vi "Check_Particle_State_NextTime_Roadblock.vi"(0 "Particle State at T":T3(array[cluster]), 1 "Torque?":bool, 2 "Torque":dbl, 3 "Rot diffusion\nfor Cargo?":bool, 5 "Tau_On":i32, 7 "Tau_Off":i32, 9 "Posi_Roadblock":dbl[][](array[numeric]), 11 "Center State at T":T1, 12 "Asymmetry (X, Y)":dbl[](array[numeric]), 13 "SD":dbl, 14 "Rot diffusion\nfor Cargo":dbl format="%#_13g") -> (4 "Particle State at T+1":T2(array[cluster]), 15 "New Center State at T":T1)   [LabVIEW 2020]
uses:
  <vilib>/gmath/statdist.llb/Normal Random.vi
  <vilib>/gmath/NI_Gmath.lvlib
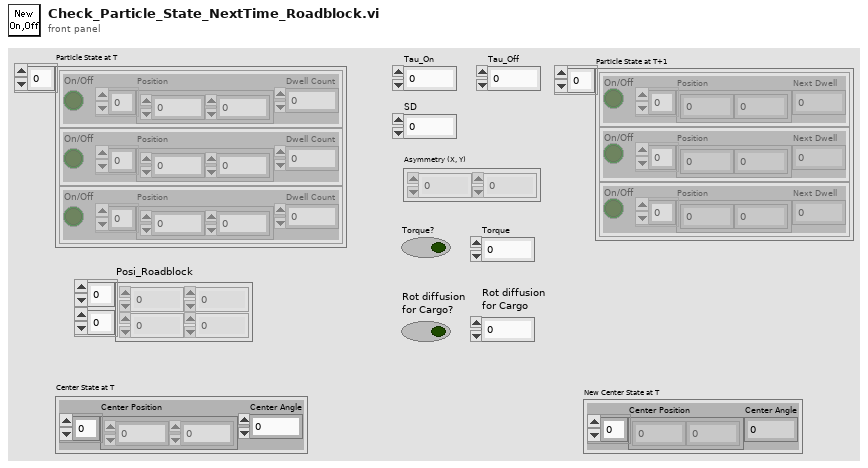
[diagram p1: front panel]
types:
  T1 = cluster{"Center Position":dbl[], "Center Angle":dbl}
  T2 = cluster{"On/Off":bool, "Position":dbl[], "Next Dwell":i32}[]
  T3 = cluster{"On/Off":bool, "Position":dbl[], "Dwell Count":i32}[]
  T4 = cluster{"On/Off":bool, "Hinderance posi":dbl[], "Next Dwell":i32}
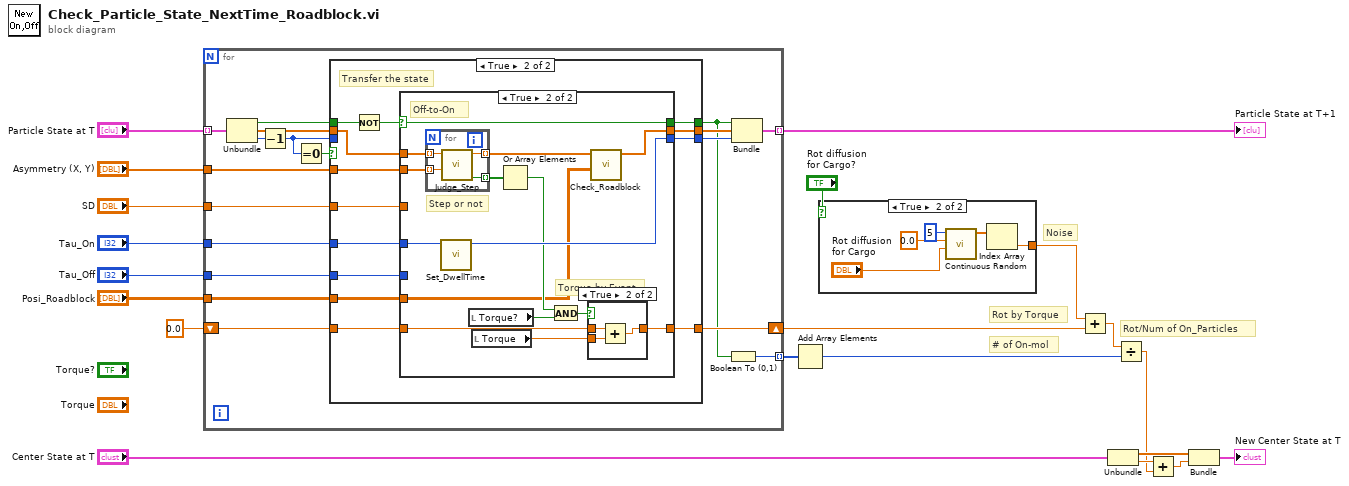
[diagram p0: block diagram]
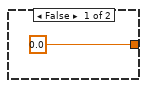
[diagram p2: hidden frame]
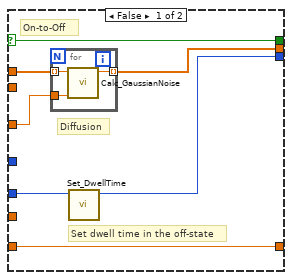
[diagram p4: hidden frame]
diagram:
  # "# of On-mol"
  # "Rot by Torque"
  # "Noise"
  # "Rot/Num of On_Particles"
  n1 = for {
    tunnel: "Particle State at T" -> [w38] mode=indexing
    tunnel: "Tau_On" -> [w32]
    tunnel: "Tau_Off" -> [w30]
    tunnel: [w29] -> w17 mode=indexing
    tunnel: "Asymmetry (X, Y)" -> [w27]
    tunnel: "SD" -> [w26]
    shift-right: [w24] -> w4
    shift-left: 0.0 -> [w25]
    tunnel: [w22] -> w13 mode=indexing
    tunnel: "Posi_Roadblock" -> [w21]
    n2 = Unbundle(w38) -> ("On/Off"=w35:bool, "Position"=w34:dbl[], "Dwell Count"=w37:i32)
    n3 = Decrement(x=w37) -> (x-1=w28:i32)
    n4 = Equal To 0?(x=w28) -> (x = 0?=w36:bool)
    n5 = case shown="TRUE" w36 {
      tunnel: w35 -> [w42 w51]
      tunnel: [w42 w47] -> w23
      tunnel: w34 -> [w41 w50]
      tunnel: [w41 w48] -> w33
      tunnel: w32 -> [_ w55]
      tunnel: [w40 w54] -> w31
      tunnel: w30 -> [_ w53]
      tunnel: w28 -> [w40 _]
      tunnel: w27 -> [_ w49]
      tunnel: w26 -> [_ w46]
      tunnel: w25 -> [w39 w44]
      tunnel: [w39 w45] -> w24
      tunnel: w21 -> [_ w43]
      frame False {
        # "Not transfering state"
      }
      frame True {
        # "Transfer the state"
        n6 = Not(x=w51) -> (.not. x?=w52:bool)
        n7 = case shown="TRUE" w52 {
          selector: w52 -> [w60 w72]
          tunnel: w55 -> [_ w80]
          tunnel: [w61 w79] -> w54
          tunnel: w53 -> [w62 _]
          tunnel: w50 -> [w59 w78]
          tunnel: w49 -> [_ w77]
          tunnel: [w58 w67] -> w48
          tunnel: [w60 w72] -> w47
          tunnel: w46 -> [w57 _]
          tunnel: w44 -> [w56 w75]
          tunnel: [w56 w76] -> w45
          tunnel: w43 -> [_ w66]
          frame False {
            # "On-to-Off"
            # "Set dwell time in the off-state"
            # "Diffusion"
            n8 = for {
              tunnel: w59 -> [w65] mode=indexing
              tunnel: [w64] -> w58 mode=indexing
              tunnel: w57 -> [w63]
              n9 = call "Calc_GaussianNoise.vi"("SD"=w63, "Start Position"=w65) -> ("Final Position"=w64:dbl)  [unwired: 9 in]
            }
            n10 = call "Set_DwellTime.vi"("Tau"=w62) -> ("Next Dwell"=w61:i32)  [unwired: 10 in]
          }
          frame True {
            # "Off-to-On"
            # "Step or not"
            # "Torque by Event"
            n11 = for {
              tunnel: w78 -> [w88] mode=indexing
              tunnel: w77 -> [w87] mode=indexing
              tunnel: [w86] -> w68 mode=indexing
              tunnel: [w85] -> w70 mode=indexing
              n12 = call "Judge_Step.vi"("Asymmetry"=w87, "Position"=w88) -> ("Off To On?"=w85:bool, "New Position"=w86:dbl)  [unwired: 8 in]
            }
            n13 = call "Set_DwellTime.vi"("Tau"=w80) -> ("Next Dwell"=w79:i32)  [unwired: 10 in]
            n14 = local read "Torque?"() -> (w74:bool)
            n15 = local read "Torque"() -> (w71:dbl)
            n16 = Or Array Elements(Boolean array=w70) -> (logical OR=w69:bool)
            n17 = And(x=w69, y=w74) -> (x .and. y?=w73:bool)
            n18 = case shown="TRUE" w73 {
              tunnel: w75 -> [w81 w83]
              tunnel: [w81 w82] -> w76
              tunnel: w71 -> [_ w84]
              frame False {
              }
              frame True {
                n19 = Add(x=w83, y=w84) -> (x+y=w82:dbl)
              }
            }
            n20 = call "Check_Roadblock.vi"("Posi_Roadblock"=w66, "New Posi"=w68) -> ("Hinderance posi"=w67:dbl[])  [unwired: 8 in, 1 out]
          }
        }
      }
    }
    n21 = Boolean To (0,1)(Boolean=w23) -> (0, 1=w22:i16)
    n22 = Bundle("On/Off"=w23, "Hinderance posi"=w33, "Next Dwell"=w31) -> (w29:T4)  [unwired: 1 in]
  }
  "Particle State at T+1" <- w17
  n23 = Add Array Elements(numeric array=w13) -> (sum=w6:i16)
  n24 = case shown="TRUE" "Rot diffusion\nfor Cargo?" {
    tunnel: [0.0 w91] -> w3
    frame False {
    }
    frame True {
      n25 = call-poly <vilib>:"Continuous Random.vi"("std"="Rot diffusion\nfor Cargo", "mean"=0.0, "samples"=5) -> ("normal random data"=w94:dbl[])  [unwired: 7 in, 1 out]
      n26 = Index Array(array=w94) -> (element=w91:dbl)  [unwired: 1 in]
    }
  }
  n27 = Add(x=w3, y=w4) -> (x+y=w2:dbl)
  n28 = Unbundle("Center State at T") -> ("Center Position"=w11:dbl[], "Center Angle"=w10:dbl)
  n29 = Divide(x=w2, y=w6) -> (x/y=w9:dbl)
  n30 = Add(x=w10, y=w9) -> (x+y=w8:dbl)
  n31 = Bundle("Center Position"=w11, w8) -> (→"New Center State at T":cluster{"Center Position":dbl[], dbl})  [unwired: 1 in]
